vi "Get All Tags.vi"(8 "error in (no error)":errorcluster, 11 "uData in":refnum<class "uData.lvclass">) -> (0 "error out":errorcluster, 2 "Map":map{string, variant}(c390), 3 "uData out":refnum<class "uData.lvclass">)   [LabVIEW 2021, in "uData.lvlib" / "uData.lvclass"]
doc: "List all tags as a map.\n\nThis method excludes the metatags are used to conserve namespaces for library-specific metatags."
uses:
  uData.lvclass
  uData.lvclass/uData.ctl
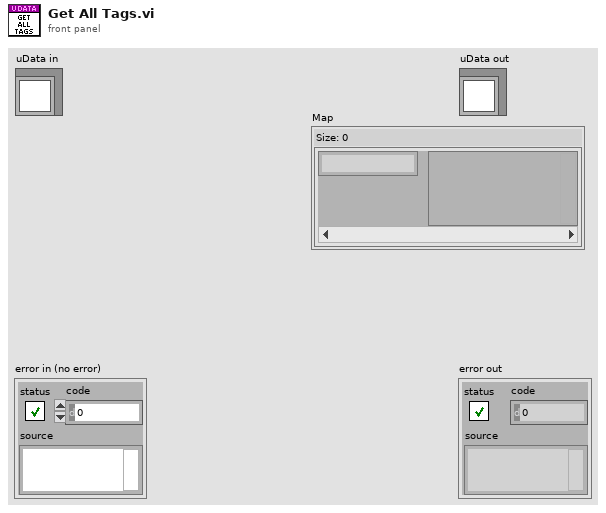
[diagram p1: front panel]
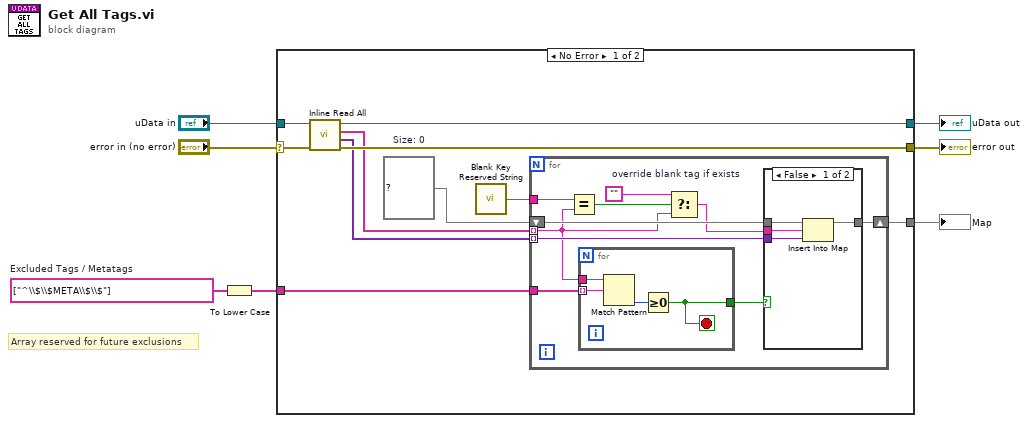
[diagram p0: block diagram]
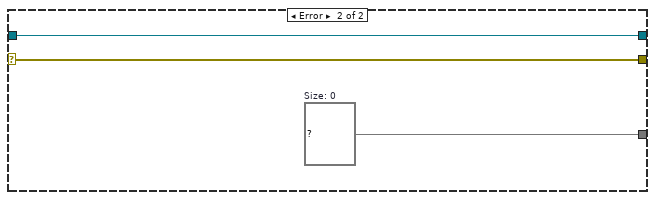
[diagram p3: hidden frame]
diagram:
  w1 = string[] ["^\\$\\$META\\$\\$"]  # Excluded Tags / Metatags
  # "Array reserved for future exclusions"
  n1 = To Lower Case(string=w1) -> (all lower case string=w2:string[])
  n2 = case shown="No Error" "error in (no error)" {
    selector: "error in (no error)" -> [w16 w39]
    tunnel: "uData in" -> [w10 w38]
    tunnel: [w11 w38] -> w6
    tunnel: [w17 w39] -> w5
    tunnel: [w12 w37] -> w3
    tunnel: w2 -> [w8 _]
    frame No Error {
      w15 = map{string, variant} {}  # Size: 0
      n3 = call "Inline Read All.vi"("error in (no error)"=w16, "uData in"=w10) -> ("error out"=w17:errorcluster, "values"=w14:variant[], "keys"=w13:string[], "uData out"=w11:refnum<class "uData.lvclass">)  [unwired: 6 in]
      n4 = call "Blank Key Reserved String.vi"() -> ("Reserved characters"=w9:string)
      n5 = for {
        shift-right: [w26] -> w12
        shift-left: w15 -> [w27]
        tunnel: w14 -> [w25] mode=indexing
        tunnel: w13 -> [w19] mode=indexing
        tunnel: w9 -> [w22]
        tunnel: w8 -> [w20]
        n6 = Equal?(x=w22, y=w19) -> (x = y?=w23:bool)
        n7 = for {
          tunnel: w20 -> [w31] mode=indexing
          tunnel: w19 -> [w30]
          tunnel: [w28] -> w18
          stop <- w28 stop-if-true
          n8 = Match Pattern(string=w30, regular expression=w31) -> (offset past match=w29:i32)  [unwired: 1 in, 3 out]
          n9 = Greater Or Equal To 0?(x=w29) -> (x >= 0?=w28:bool)
        }
        n10 = Select "override blank tag if exists"(t="", s=w23, f=w19) -> (s? t:f=w24:string)
        n11 = case shown="False" w18 {
          tunnel: w27 -> [w35 w36]
          tunnel: [w34 w36] -> w26
          tunnel: w25 -> [w33 _]
          tunnel: w24 -> [w32 _]
          frame False {
            n12 = Insert Into Map(map in=w35, key=w32, value=w33) -> (map out=w34:map{string, variant})  [unwired: 2 out]
          }
          frame True {
            # "Exclude tag"
          }
        }
      }
    }
    frame Error {
      w37 = map{string, variant} {}  # Size: 0
    }
  }
  "error out" <- w5
  "uData out" <- w6
  "Map" <- w3
